vi "Safety Trigger.vi"(8 "error in (no error)":errorcluster, 10 "Safety Trigger":bool) -> (0 "error out":errorcluster, 2 "Trigger State":bool)   [LabVIEW 2017, in "Haptic Prog Interface.lvlib"]
doc: "Returns the forces of the haptic pen in N.\n\n<b>Position:</b> Returns a cluster of the x, y, and z forces on the pen (in units of N)."
uses:
  Haptic Prog Interface.lvlib
  Haptic-Programming-Interface/src/x64/Debug/Haptic Programming Interface.dll
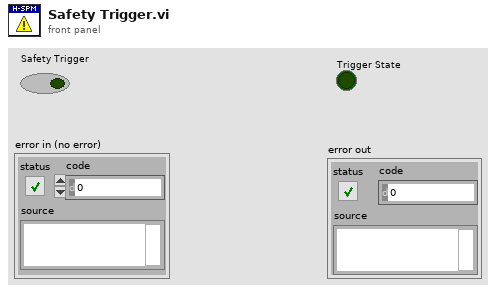
[diagram p1: front panel]
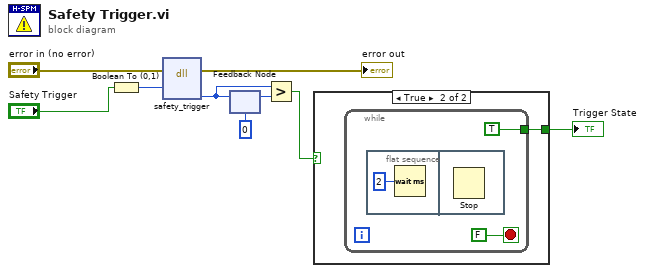
[diagram p0: block diagram]
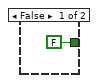
[diagram p2: hidden frame]
diagram:
  n1 = Boolean To (0,1)(Boolean="Safety Trigger") -> (0, 1=w7:i16)
  n2 = dll-call lib="C:/Users/freem/Documents/GitHub/HapticSPM/Haptic-Programming-Interface/src/x64/Debug/Haptic Programming Interface.dll" fn="safety_trigger"(error in="error in (no error)", "input"=w7) -> (error out=→"error out":errorcluster, "output"=w1:i32)  [unwired: 5 in, 1 out]
  n3 = feedback-in #1(w1) -> ()
  n4 = feedback #1(0) -> (w4:i32)
  n5 = Greater?(x=w1, y=w4) -> (0:w3:bool)
  n6 = case shown="True" w3 {
    tunnel: [FALSE w11] -> w2
    frame False {
    }
    frame True {
      n7 = while {
        tunnel: [TRUE] -> w11
        stop <- FALSE stop-if-true
        n8 = flat-sequence {
          frame #0 {
            n9 = Wait (ms)(milliseconds to wait=u32 2) -> ()  [unwired: 1 out]
          }
          frame #1 {
            n10 = Stop() -> ()  [unwired: 1 in]
          }
        }
      }
    }
  }
  "Trigger State" <- w2
